vi "Command (write) - PR.vi"(7 "timeout ms (100)":i32=100, 8 "error in (no error)":errorcluster, 9 "Protocol Setting":string, 10 "IP":string, 11 "connection ID in":refnum<k16>) -> (0 "error out":errorcluster, 3 "connection ID out":refnum<k16>)   [LabVIEW 2016, in "SMD-7615.lvlib" / "eSCL.lvlib"]
doc: "PR - Protocol\nSets or requests the serial communication protocol settings. Sets or requests the serial communication protocol\nsettings. There are a number of settings that can be turned on or off in the PR command. Each setting is\nassigned a bit in a 9 - bit binary word. The parameter of the PR command is the decimal equivalent of this word. If you send the PR command without a parameter the drive will respond with the decimal equivalent of the word as well. The different protocol settings and their bit assignments are shown below."
uses:
  eSCL.lvlib
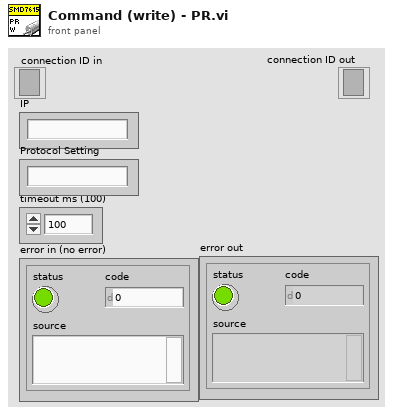
[diagram p1: front panel]
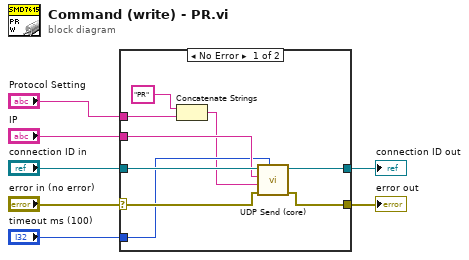
[diagram p0: block diagram]
diagram:
  n1 = case shown="No Error" "error in (no error)" {
    selector: "error in (no error)" -> [w16 w17]
    tunnel: "connection ID in" -> [w15 w18]
    tunnel: [w10 w18] -> w5
    tunnel: [w9 w17] -> w4
    tunnel: "IP" -> [w14 _]
    tunnel: "timeout ms (100)" -> [w13 _]
    tunnel: "Protocol Setting" -> [w11 _]
    frame No Error {
      n2 = Concatenate Strings("PR" ("Data"), w11) -> (w8:string)
      n3 = call "UDP Send (core).vi"("timeout ms (100)"=w13, "error in (no error)"=w16, "Data"=w8, "IP"=w14, "connection ID in"=w15) -> ("error out"=w9:errorcluster, "connection ID out"=w10:refnum<k16>)  [unwired: 5 in]
    }
    frame Error {
    }
  }
  "connection ID out" <- w5
  "error out" <- w4
